vi "LECTURA&ESCRITURA_ARDUINO.vi"() -> ()   [LabVIEW 2021]
uses:
  <vilib>/Instr/_visa.llb/VISA Configure Serial Port (Instr).vi
panel:
  out "PIN 3 PWM":i32
  in  "stop":bool
  out "A0":i32
  out "Waveform Chart":dynamicdata(graph)
  in  "STEP":dbl(slide) scale=0.0..100.0
  in  "PUERTO COM \nEN ARDUINO":refnum<visa-resource-name>
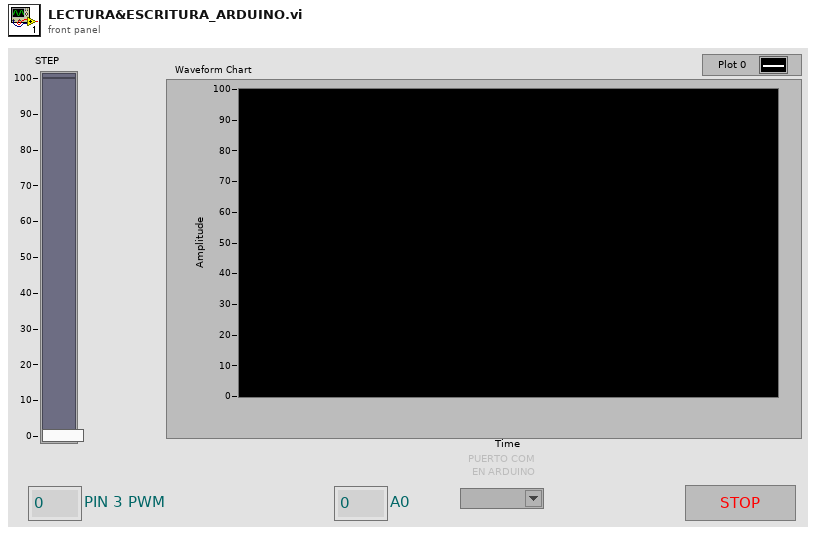
[diagram p1: front panel]
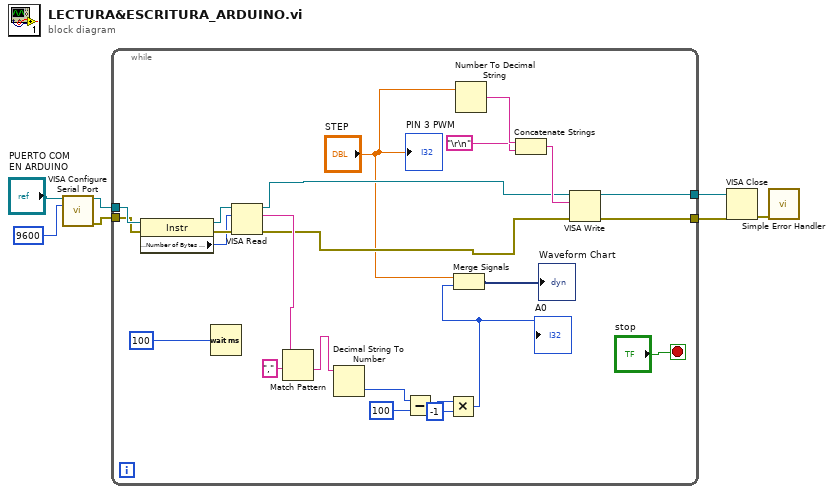
[diagram p0: block diagram]
diagram:
  n1 = call-poly "VISA Configure Serial Port"("VISA resource name"="PUERTO COM \nEN ARDUINO", "baud rate (9600)"=u32 9600) -> ("VISA resource name out"=w4:refnum<visa-resource-name>, "error out"=w3:errorcluster)  [unwired: 12 in]
  n2 = while {
    tunnel: w4 -> [w18]
    tunnel: w3 -> [w17]
    tunnel: [w16] -> w2
    tunnel: [w15] -> w1
    stop <- "stop" stop-if-true
    n3 = property class="Instr"(reference=w18, error in=w17) -> (reference out=w30:refnum<visa-resource-name>, error out=w29:errorcluster, "Serial Settings:Number of Bytes at Serial Port"=w28:u32)
    n4 = Wait (ms)(milliseconds to wait=u32 100) -> ()  [unwired: 1 out]
    n5 = VISA Read(VISA resource name=w30, byte count=w28, error in (no error)=w29) -> (VISA resource name out=w21:refnum<visa-resource-name>, read buffer=w27:string, error out=w20:errorcluster)  [unwired: 1 out]
    n6 = Match Pattern(string=w27, regular expression=",") -> (after substring=w25:string)  [unwired: 1 in, 3 out]
    n7 = Decimal String To Number(string=w25) -> (number=w12:i32)  [unwired: 2 in, 1 out]
    n8 = Subtract(x=w12, y=100) -> (x-y=w10:i32)
    n9 = Multiply(x=w10, y=-1) -> (x*y=w8:i32)
    "A0" <- w8
    n10 = Merge Signals("STEP", w8) -> (→"Waveform Chart":dynamicdata)
    n11 = Number To Decimal String(number="STEP") -> (decimal integer string=w23:string)  [unwired: 1 in]
    n12 = Concatenate Strings(w23, "\r\n") -> (w24:string)
    n13 = VISA Write(VISA resource name=w21, write buffer=w24, error in (no error)=w20) -> (VISA resource name out=w16:refnum<visa-resource-name>, error out=w15:errorcluster)  [unwired: 1 out]
    "PIN 3 PWM" <- "STEP"
  }
  n14 = VISA Close(VISA resource name=w2, error in (no error)=w1) -> (error out=w6:errorcluster)
  n15 = call <vilib>:"Simple Error Handler.vi"("error in (no error)"=w6) -> ()  [unwired: 4 in, 5 out]
